vi "Get Root.vi"(8 "error in (no error)":errorcluster, 11 "PathTree in":refnum<class "PathTree.lvclass">) -> (0 "error out":errorcluster, 2 "Root":refnum<class "PathTreeNode.lvclass">, 3 "PathTree out":refnum<class "PathTree.lvclass">)   [LabVIEW 2020, in "PathTree.lvlib" / "PathTree.lvclass"]
uses:
  PathTree.lvclass
  PathTreeNode/PathTreeNode.lvclass
  PathTree.lvclass/PathTree.ctl
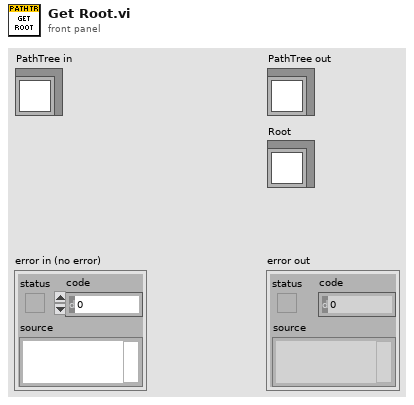
[diagram p1: front panel]
types:
  T1 = typedef "Advanced Structures.lvlib/PathTree.lvclass/Ref Data.ctl" = cluster{"Root":refnum<class>}
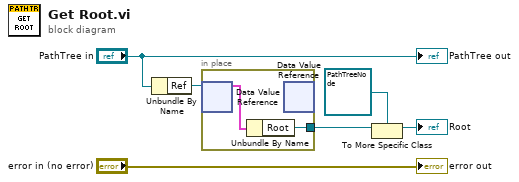
[diagram p0: block diagram]
diagram:
  n1 = Unbundle By Name("PathTree in") -> ("Ref"=w5:refnum<data-value>)
  n2 = in-place {
    in-place-border: [w7] -> w3
    n3 = in-place-dvr #1(w5) -> (w8:T1)  [unwired: 1 out]
    n4 = Unbundle By Name(w8) -> ("Root"=w7:refnum<class>)
    n5 = in-place-dvr #1() -> ()  [unwired: 1 in, 2 out]
  }
  n6 = To More Specific Class(target class=refnum<class "PathTreeNode.lvclass"> refnum ("Advanced Structures.lvlib:PathTreeNode.lvclass"), reference=w3) -> (specific class reference=→"Root":refnum<class "PathTreeNode.lvclass">)  [unwired: 1 in, 1 out]
  "error out" <- "error in (no error)"
  "PathTree out" <- "PathTree in"
